vi "ConvertDD2DMS.vi"(7 "Type":bool=TRUE, 8 "error in":errorcluster, 10 "Decimal String":string, 11 "Degree Decimal":dbl format="%.6f") -> (0 "error out":errorcluster, 1 "Seconds":dbl, 2 "Minutes":dbl, 3 "Degrees":dbl, 5 "NE?":bool)   [LabVIEW 2010]
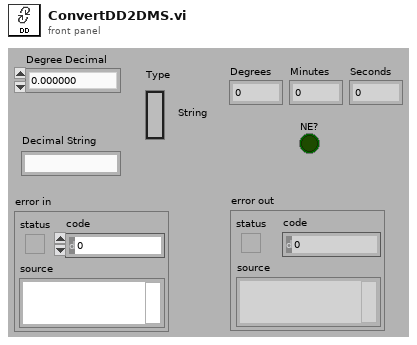
[diagram p1: front panel]
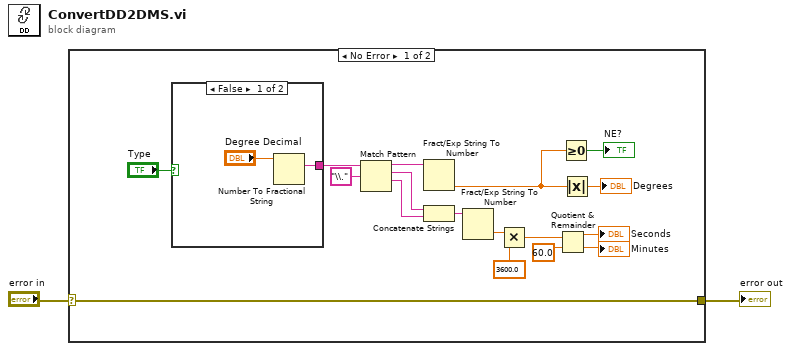
[diagram p0: block diagram]
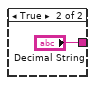
[diagram p2: hidden frame]
diagram:
  n1 = case shown="No Error" "error in" {
    selector: "error in" -> [w18 w23]
    tunnel: [w18 w23] -> w1
    frame No Error {
      n2 = case shown="False" "Type" {
        tunnel: [w20 "Decimal String"] -> w17
        frame False {
          n3 = Number To Fractional String(number="Degree Decimal") -> (F-format string=w20:string)  [unwired: 3 in]
        }
        frame True {
        }
      }
      n4 = Match Pattern(string=w17, regular expression="\\.") -> (before substring=w15:string, match substring=w11:string, after substring=w10:string)  [unwired: 1 in, 1 out]
      n5 = Fract/Exp String To Number(string=w15) -> (number=w4:dbl)  [unwired: 3 in, 1 out]
      n6 = Concatenate Strings(w11, w10) -> (w12:string)
      n7 = Fract/Exp String To Number(string=w12) -> (number=w9:dbl)  [unwired: 3 in, 1 out]
      n8 = Multiply(x=w9, y=3600.0) -> (x*y=w7:dbl)
      n9 = Quotient & Remainder(x=w7, y=60.0) -> (x-y*floor(x/y)=→"Seconds":dbl, floor(x/y)=→"Minutes":dbl)
      n10 = Greater Or Equal To 0?(x=w4) -> (x >= 0?=→"NE?":bool)
      n11 = Absolute Value(x=w4) -> (abs(x)=→"Degrees":dbl)
    }
    frame Error {
    }
  }
  "error out" <- w1
